vi "Pattern_Gen_Opcode.vi"() -> ()   [LabVIEW 2016]
uses:
  Classes/Config_Read/Config_Read_BML.lvclass
  Classes/BML_DigiPattern_Generator/DigiPattern_Generator.lvclass
  Classes/BML_Frame_Write_Opcode/BML_Frame_Write_Opcode.lvclass
  C:/Users/8135/Desktop/BML_Pattern_Gen/BeamLink_Pattern_Gen/BML_Pattern_Gen_Refactor/Classes/BML_Frame_Root/BML_Frame_Root.lvclass
  Classes/BML_Frame_RW/BML_Frame_RW.lvclass
  Classes/BML_Frame_Read/BML_Frame_Read.lvclass
  Classes/BML_Frame_SetID/BML_Frame_SetID.lvclass
  Classes/Config_Read/RW_Option.ctl
  Classes/Config_Read/BurstLength.ctl
  Classes/Config_Read/OperationMode.ctl
  Classes/Config_Read/Frame_Data.ctl
panel:
  in  "num of delay cycles before read capture":i8=1
  in  "Timeset between frms":u32=40
  out "error out":errorcluster
  in  "PinMap":path
  in  "ChipID":u8=1
  in  "Config Path":path
  in  "error in (no error)":errorcluster
  # "Version 1.2.2\nAdd Pattern Name check, which should be the same as CSV file name\nAdd delay cycle settings"
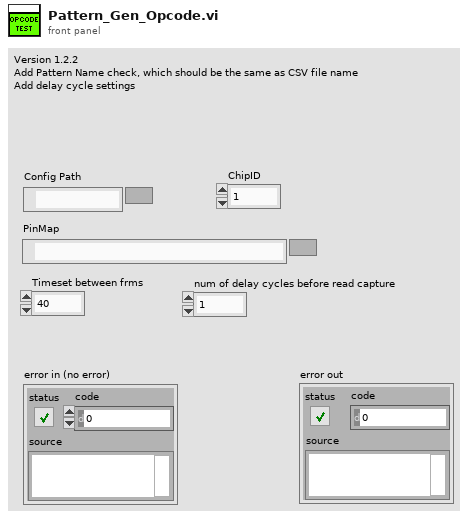
[diagram p1: front panel]
types:
  T1 = typedef "Config_Read_BML.lvclass/Frame_Data.ctl" = cluster{"Pattern_Name":string, "Operation Mode":T2, "BurstLength":T3, "FSN":u8, "Start_Addr":u16, "Data":u8[], "R/W?":T4, "Opcode":string[], "ChipID":u8, "num of wait cycle of read":i8}
  T2 = typedef "Config_Read_BML.lvclass/OperationMode.ctl" = enum8{"Normal", "ImmeEffect", "InitSlaveID", "LoadData"}
  T3 = typedef "Config_Read_BML.lvclass/BurstLength.ctl" = enum8{"0", "2", "3", "4", "5", "8", "16", "32"}
  T4 = typedef "Config_Read_BML.lvclass/RW_Option.ctl" = enum16{"Read", "Write", "R/W"}
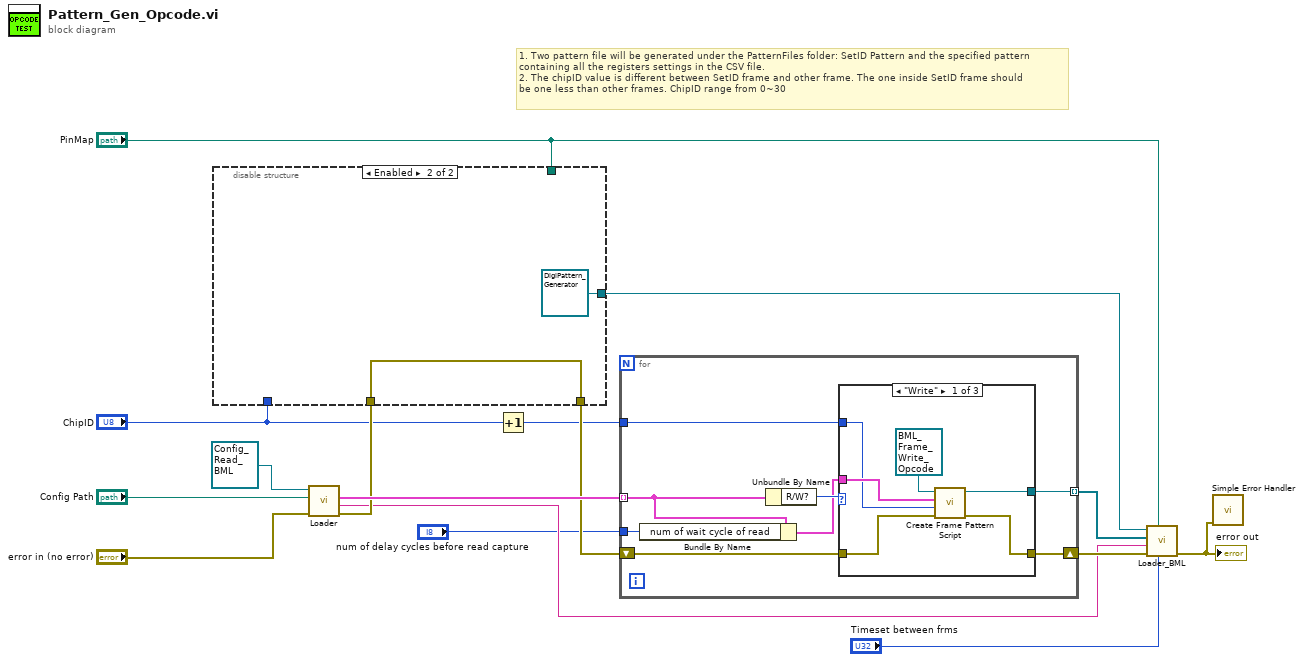
[diagram p0: block diagram]
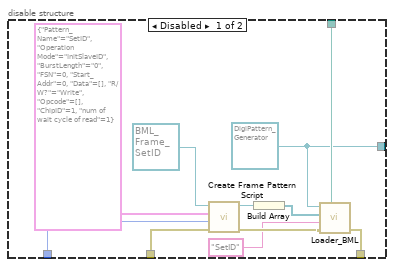
[diagram p2: hidden frame]
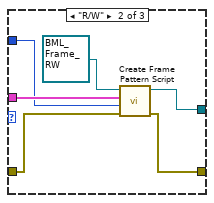
[diagram p3: hidden frame]
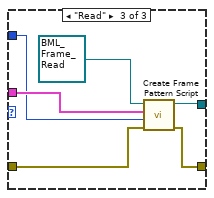
[diagram p4: hidden frame]
diagram:
  # "1. Two pattern file will be generated under the PatternFiles folder: SetID Pattern and the specified pattern\ncontaining all the registers settings in the CSV file.\n2. The chipID value is different between SetID frame and other frame. The one inside SetID frame should \nbe one less than other frames. ChipID range from 0~30"
  n1 = call "Loader.vi"("error in (no error)"="error in (no error)", "Path"="Config Path", "Config_Read.lvclass"=refnum<class "Config_Read_BML.lvclass"> refnum) -> ("error out"=w12:errorcluster, "Pattern_Name"=w5:string, "FRM_Data_Array"=w13:T1[])  [unwired: 5 in, 1 out]
  n2 = disable-structure shown="Enabled" {
    disable-tunnel: w12 -> [w25 w28]
    disable-tunnel: [w24 w28] -> w11
    disable-tunnel: "ChipID" -> [w21 _]
    disable-tunnel: "PinMap" -> [w18 _]
    disable-tunnel: [w17 refnum<class "DigiPattern_Generator.lvclass"> refnum ("BML_DigiPattern_Generator.lvclass")] -> w4
    frame Disabled {
      w17 = refnum<class "DigiPattern_Generator.lvclass"> refnum ("BML_DigiPattern_Generator.lvclass")
      n3 = call-dynamic "Create Frame Pattern Script.vi"("error in (no error)"=w25, "ChipID"=w21, "Frame_Data"=T1 {"Pattern_Name"="SetID", "Operation Mode"=enum."InitSlaveID", "BurstLength"=enum."0", "FSN"=0, "Start_Addr"=0, "Data"=[], "R/W?"=enum."Write", "Opcode"=[], "ChipID"=1, "num of wait cycle of read"=1}, "BML_Frame_SetID in"=refnum<class "BML_Frame_SetID.lvclass"> refnum ("BML_Frame_SetID.lvclass")) -> ("error out"=w23:errorcluster, "BML_Frame_SetID out"=w20:refnum<class "BML_Frame_SetID.lvclass">)  [unwired: 6 in]
      n4 = Build Array(w20) -> (w19:refnum<class "BML_Frame_SetID.lvclass">[])
      n5 = call "Loader_BML.vi"("PinMap"=w18, "error in (no error)"=w23, "Pattern Name"="SetID", "BML Frame Array"=w19, "BML_DigiPattern_Generator.lvclass"=w17) -> ("error out"=w24:errorcluster)  [unwired: 5 in, 1 out]
    }
    frame Enabled {
    }
  }
  n6 = Increment(x="ChipID") -> (x+1=w9:u8)
  n7 = for {
    tunnel: w13 -> [w32] mode=indexing
    tunnel: w9 -> [w35]
    shift-right: [w34] -> w8
    shift-left: w11 -> [w36]
    tunnel: [w33] -> w7 mode=indexing
    tunnel: "num of delay cycles before read capture" -> [w30]
    n8 = Bundle By Name(cluster=w32, "num of wait cycle of read"=w30) -> (w31:T1)
    n9 = Unbundle By Name(w32) -> ("R/W?"=w37:T4)
    n10 = case shown="\"Write\"" w37 {
      tunnel: w36 -> [w42 w46 w53]
      tunnel: w31 -> [w43 w48 w51]
      tunnel: w35 -> [w41 w47 w50]
      tunnel: [w40 w44 w54] -> w33
      tunnel: [w39 w45 w52] -> w34
      frame "Write" {
        n11 = call-dynamic "Create Frame Pattern Script.vi"("error in (no error)"=w42, "ChipID"=w41, "Frame_Data"=w43, "BML_Frame_Write_Opcode in"=refnum<class "BML_Frame_Write_Opcode.lvclass"> refnum ("BML_Frame_Write_Opcode.lvclass")) -> ("error out"=w39:errorcluster, "BML_Frame_Write_Opcode out"=w40:refnum<class "BML_Frame_Write_Opcode.lvclass">)  [unwired: 6 in]
      }
      frame "R/W" {
        n12 = call-dynamic "Create Frame Pattern Script.vi"("error in (no error)"=w46, "ChipID"=w47, "Frame_Data"=w48, "BML_Frame_RW in"=refnum<class "BML_Frame_RW.lvclass"> refnum ("BML_Frame_RW.lvclass")) -> ("error out"=w45:errorcluster, "BML_Frame_RW out"=w44:refnum<class "BML_Frame_RW.lvclass">)  [unwired: 6 in]
      }
      frame "Read" {
        n13 = call-dynamic "Create Frame Pattern Script.vi"("error in (no error)"=w53, "ChipID"=w50, "Frame_Data"=w51, "BML_Frame_Read in"=refnum<class "BML_Frame_Read.lvclass"> refnum ("BML_Frame_Read.lvclass")) -> ("error out"=w52:errorcluster, "BML_Frame_Read out"=w54:refnum<class "BML_Frame_Read.lvclass">)  [unwired: 6 in]
      }
    }
  }
  n14 = call "Loader_BML.vi"("Timeset between frms"="Timeset between frms", "PinMap"="PinMap", "error in (no error)"=w8, "Pattern Name"=w5, "BML Frame Array"=w7, "BML_DigiPattern_Generator.lvclass"=w4) -> ("error out"=w3:errorcluster)  [unwired: 4 in, 1 out]
  "error out" <- w3
  n15 = call <vilib>:"Simple Error Handler.vi"("error in (no error)"=w3) -> ()  [unwired: 4 in, 5 out]
